vi "Status Update.vi"(8 "error in (no error)":errorcluster, 9 "Status":string, 10 "Name":string, 11 "Server in":refnum<class "Server.lvclass">) -> (0 "error out":errorcluster, 3 "Server out":refnum<class "Server.lvclass">)   [LabVIEW 2018, in "Server.lvlib" / "Server.lvclass"]
uses:
  Server.lvclass
  Server.lvclass/Server.ctl
  Chat Window Model/Chat Window Model Messages/Update Status Log Msg/Update Status Log Msg.lvclass/Update Status Log Msg.ctl
  <vilib>/ActorFramework/Message Enqueuer/Message Enqueuer.lvclass/Message Enqueuer.ctl
  <vilib>/ActorFramework/Message Enqueuer/Enqueue.vi
  Chat Window Model/Chat Window Model Messages/Update Status Log Msg/Update Status Log Msg.lvclass
  C:/Program Files (x86)/National Instruments/LabVIEW 2018/vi.lib/ActorFramework/Message/Message.lvclass
  <vilib>/ActorFramework/Message Priority Queue/Priority Enqueue.vi
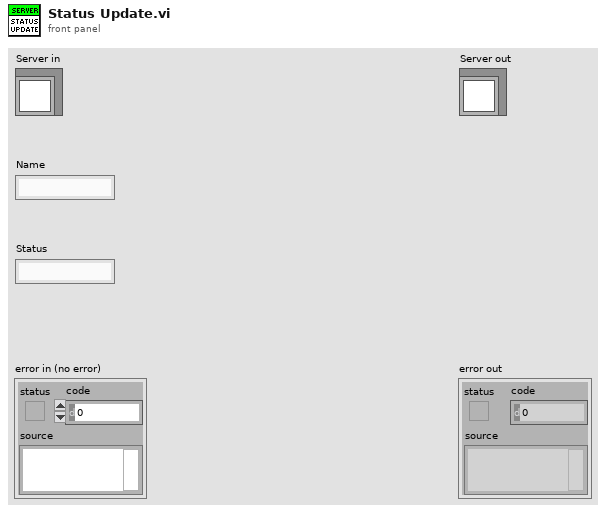
[diagram p1: front panel]
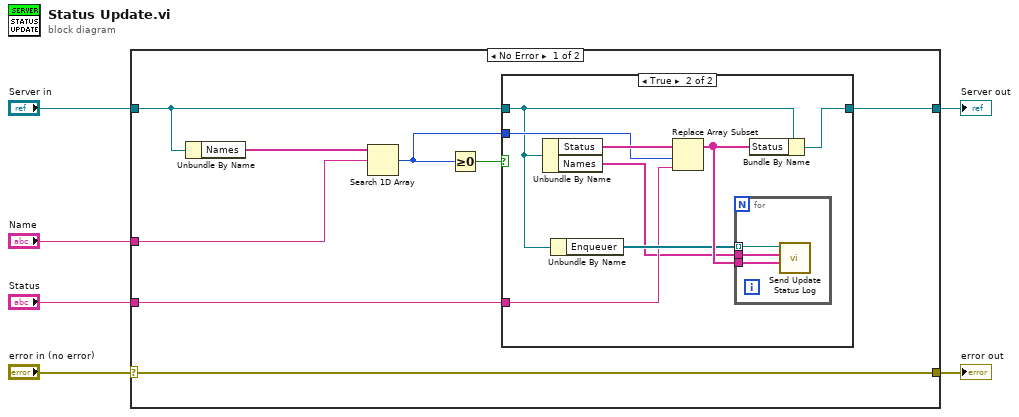
[diagram p0: block diagram]
diagram:
  n1 = case shown="No Error" "error in (no error)" {
    selector: "error in (no error)" -> [w14 w28]
    tunnel: [w14 w28] -> w5
    tunnel: [w12 w27] -> w3
    tunnel: "Server in" -> [w13 w27]
    tunnel: "Status" -> [w7 _]
    tunnel: "Name" -> [w10 _]
    frame No Error {
      n2 = Unbundle By Name(w13) -> ("Names"=w11:string[])
      n3 = Search 1D Array(1D array=w11, element=w10) -> (index of element=w9:i32)  [unwired: 1 in]
      n4 = Greater Or Equal To 0?(x=w9) -> (x >= 0?=w8:bool)
      n5 = case shown="True" w8 {
        tunnel: w13 -> [w15 w19]
        tunnel: w9 -> [_ w22]
        tunnel: [w15 w21] -> w12
        tunnel: w7 -> [_ w17]
        frame False {
        }
        frame True {
          n6 = Unbundle By Name(w19) -> ("Status"=w23:string[], "Names"=w16:string[])
          n7 = Unbundle By Name(w19) -> ("Enqueuer"=w18:refnum<class "Message Enqueuer.lvclass">[])
          n8 = Replace Array Subset(array=w23, new element=w17, index=w22) -> (w20:string[])
          n9 = for {
            tunnel: w20 -> [w25]
            tunnel: w18 -> [w26] mode=indexing
            tunnel: w16 -> [w24]
            n10 = call "Send Update Status Log.vi"("Status List"=w25, "Names"=w24, "Message Enqueuer"=w26) -> ()  [unwired: 7 in, 2 out]
          }
          n11 = Bundle By Name(cluster=w19, "Status"=w20) -> (w21:refnum<class "Server.lvclass">)
        }
      }
    }
    frame Error {
    }
  }
  "error out" <- w5
  "Server out" <- w3
